vi "Begin.vi"(8 "error in":errorcluster) -> (0 "error out":errorcluster)   [LabVIEW 2014]
doc: "Called before other user functions, this VI is expected to open initial I/O refnums, load in file data, and do all program initialization. Notice that the <B>error out</B> terminal is simply used for data flow. Wiring it to other structures or subVIs ensures that this VI runs first."
uses:
  <vilib>/Rock Robotics/SystemInterfaces/DIO/FPGA_DIOPWMChannel.ctl
  <vilib>/Rock Robotics/WPI/SafetyOutput/WPI_SafetyOutputConfigMenu.ctl
  <vilib>/Rock Robotics/WPI/DriverStation/WPI_DriverStationRobotMode2.ctl
  <vilib>/Rock Robotics/WPI/Joystick/WPI_JoystickDeviceEnum.ctl
  <vilib>/Rock Robotics/WPI/Solenoid/WPI_SolenoidChannel.ctl
  <vilib>/Rock Robotics/SystemInterfaces/DIO/FPGA_DIOChannel.ctl
  <vilib>/Rock Robotics/WPI/Encoder/WPI_EncoderType.ctl
  <vilib>/Rock Robotics/SystemInterfaces/AI/FPGA_AIGyroChannel.ctl
  <vilib>/Rock Robotics/SystemInterfaces/Typedef/FPGA_TypedefAnalogModule.ctl
  <vilib>/Rock Robotics/SystemInterfaces/AI/FPGA_AIChannel.ctl
  <vilib>/Rock Robotics/SystemInterfaces/Typedef/FPGA_TypedefDigitalModule.ctl
  <vilib>/Rock Robotics/SystemInterfaces/Typedef/FPGA_TypedefAnalogModuleForGyro.ctl
  <vilib>/Rock Robotics/WPI/RobotDrive/WPI_RobotDriveOpen2MotorWithTalon.vi
  Robot Global Data.vi
  <vilib>/Rock Robotics/Network Tables/SD Write String Array.vi
  <vilib>/Rock Robotics/WPI/MotorControl/WPI_MotorControlOpen Victor.vi
  <vilib>/Rock Robotics/WPI/Solenoid/WPI_SolenoidOpenDouble.vi
  <vilib>/Rock Robotics/WPI/Counter/WPI_CounterDigitalInputToDigitalSource.vi
  <vilib>/Rock Robotics/WPI/Switch/WPI_SwitchOpenLimit.vi
  <vilib>/Rock Robotics/WPI/Accelerometer/InternalAccelerometer/WPI_AccelerometerInternalOpen.vi
  <vilib>/Rock Robotics/WPI/Camera/WPI_CameraDevRef.ctl
  <vilib>/Rock Robotics/WPI/Ultrasonic/WPI_SonarMB1010AnalogOpen.vi
  <vilib>/Rock Robotics/WPI/Ultrasonic/WPI_SonarMB1010AnalogRefNum Registry Set.vi
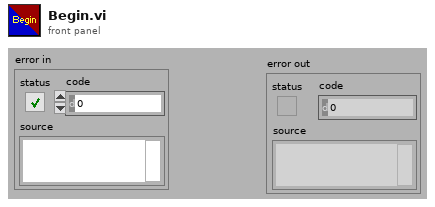
[diagram p1: front panel]
types:
  T1 = typedef "FPGA_TypedefAnalogModuleForGyro.ctl" = enum16{"Controller 1"}
  T2 = typedef "FPGA_AIGyroChannel.ctl" = enum8{"AI 0", "AI 1", "Invalid"}
  T3 = typedef "FPGA_AIChannel.ctl" = enum8{"AI 0", "AI 1", "AI 2", "AI 3", "AI MXP 0", "AI MXP 1", "AI MXP 2", "AI MXP 3", "Invalid"}
  T4 = typedef "FPGA_TypedefAnalogModule.ctl" = enum16{"Controller 1"}
  T5 = typedef "FPGA_TypedefDigitalModule.ctl" = enum16{"Controller 1"}
  T6 = typedef "WPI_EncoderType.ctl" = enum16{"1x", "2x", "4x"}
  T7 = typedef "FPGA_DIOChannel.ctl" = enum8{"DIO 0", "DIO 1", "DIO 2", "DIO 3", "DIO 4", "DIO 5", "DIO 6", "DIO 7", "DIO 8", "DIO 9", "DIO MXP 0", "DIO MXP 1", "DIO MXP 2", "DIO MXP 3", "DIO MXP 4", "DIO MXP 5", "DIO MXP 6", "DIO MXP 7", "DIO MXP 8", "DIO MXP 9", "DIO MXP 10", "DIO MXP 11", "DIO MXP 12", "DIO MXP 13", "DIO MXP 14", "DIO MXP 15", "Invalid"}
  T8 = typedef "WPI_SolenoidChannel.ctl" = enum8{"Solenoid 0", "Solenoid 1", "Solenoid 2", "Solenoid 3", "Solenoid 4", "Solenoid 5", "Solenoid 6", "Solenoid 7", "Invalid"}
  T9 = typedef "FPGA_DIOPWMChannel.ctl" = enum8{"PWM 0", "PWM 1", "PWM 2", "PWM 3", "PWM 4", "PWM 5", "PWM 6", "PWM 7", "PWM 8", "PWM 9", "PWM MXP 0", "PWM MXP 1", "PWM MXP 2", "PWM MXP 3", "PWM MXP 4", "PWM MXP 5", "PWM MXP 6", "PWM MXP 7", "PWM MXP 8", "PWM MXP 9", "Invalid"}
  T10 = typedef "WPI_JoystickDeviceEnum.ctl" = enum16{"USB 0", "USB 1", "USB 2", "USB 3", "USB 4", "USB 5"}
  T11 = typedef "WPI_DriverStationRobotMode2.ctl" = enum16{"Autonomous Disabled", "Autonomous Enabled", "Teleop Disabled", "Teleop Enabled", "Disconnected", "Finish", "Test Disabled", "Test Enabled", "Emergency Stopped"}
  T12 = typedef "WPI_SafetyOutputConfigMenu.ctl" = enum16{"Enable", "Disable"}
  T13 = typedef "WPI_CameraDevRef.ctl" = cluster{"Camera Address":string, "CameraStatus":errorcluster}
  T14 = typedef "WPI_PotentiometerDevRef.ctl" = cluster{"DevStatus":errorcluster, "Controller":T4, "Analog Channel":T3, "Invert Output":bool}
  T15 = typedef "WPI_GyroDevRef.ctl" = cluster{"DevStatus":errorcluster, "Analog Module":T4, "Analog Channel":T3, "Offset":dbl, "Gain (VoltsPerDegree/Second)":dbl}
  T16 = typedef "WPI_JoystickDevRef.ctl" = cluster{"Device":T10}
  T17 = typedef "WPI_RobotDriveDevRef.ctl" = cluster{"DevStatus":errorcluster, "Motors[]":T18[], "Square Inputs":bool, "Max Output":dbl}
  T18 = typedef "WPI_MotorControlDeviceRef.ctl" = cluster{"DeviceStatus":errorcluster, "Type":T19, "PWM":cluster{"Controller":T5, "PWM Channel":T9, "DeadBand":T20}, "CAN":cluster{"Device Number":u8, "Control Mode":T21, "Semaphore":T22, "Max Vout":dbl, "TalonSRX Control Mode":T23}, "Invert":bool, "TransformRef":T24, "InvTransformRef":T24}
  T19 = typedef "WPI_MotorControlType.ctl" = enum16{"PWM", "CAN", "CANTalonSRX"}
  T20 = typedef "WPI_PWMDeadband.ctl" = cluster{"Name":string, "maxPositivePwm":i32, "minPositivePwm":i32, "centerPwm":i32, "maxNegativePwm":i32, "minNegativePwm":i32, "angularRange":u16}
  T21 = typedef "WPI_CANJaguar_ControlMode.ctl" = enum8{"Percent VBus", "Current", "Speed", "Position", "Voltage"}
  T22 = typedef "Semaphore RefNum" = refnum<k1>
  T23 = typedef "WPI_CANTalonSRX_APIControlMode.ctl" = enum8{"Percent VBus", "Speed", "Position", "Slave", "Unchanged / Invalid"}
  T24 = typedef "WPI_PWMTransform_ConPane.ctl" = refnum<vi>
  T25 = typedef "WPI_DigitalInputDevRef.ctl" = cluster{"DevStatus":errorcluster, "DIO Channel":T7, "Controller":T5}
  T26 = typedef "FPGA_CounterEncoderSourceConvertionLVSourceType.ctl" = cluster{"DevStatus":errorcluster, "AnalogTriggerMode?":bool, "DigitalMode":cluster{"Controller":T5, "DIO Channel":T27}, "AnalogTriggerMode":cluster{"AnalogTriggerIndex":T28, "OutputType":T29}}
  T27 = typedef "FPGA_DIODigitalSourceChannel.ctl" = enum8{"DIO 0", "DIO 1", "DIO 2", "DIO 3", "DIO 4", "DIO 5", "DIO 6", "DIO 7", "DIO 8", "DIO 9", "DIO MXP 0", "DIO MXP 1", "DIO MXP 2", "DIO MXP 3", "DIO MXP 4", "DIO MXP 5", "DIO MXP 6", "DIO MXP 7", "DIO MXP 8", "DIO MXP 9", "DIO MXP 10", "DIO MXP 11", "DIO MXP 12", "DIO MXP 13", "DIO MXP 14", "DIO MXP 15", "Disabled"}
  T28 = typedef "FPGA_AnalogTriggerIndex.ctl" = enum8{"Trig 0", "Trig 1", "Trig 2", "Trig 3", "Trig 4", "Trig 5", "Trig 6", "Trig 7", "Invalid"}
  T29 = typedef "FPGA_AnalogTriggerOutType.ctl" = enum16{"InWindow", "TriggerState", "Rising", "Falling"}
  T30 = typedef "WPI_EncoderDevRef.ctl" = cluster{"DevStatus":errorcluster, "EncoderIndex":T31, "CounterIndex":T32, "DistancePerCount":dbl, "Decoding Type":T6}
  T31 = typedef "FPGA_EncoderIdx.ctl" = enum8{"Enc 0", "Enc 1", "Enc 2", "Enc 3", "Enc 4", "Enc 5", "Enc 6", "Enc 7", "Invalid"}
  T32 = typedef "FPGA_CounterCtrSystemIndex.ctl" = enum8{"Ctr 0", "Ctr 1", "Ctr 2", "Ctr 3", "Ctr 4", "Ctr 5", "Ctr 6", "Ctr 7", "Invalid"}
  T33 = typedef "WPI_AccelerometerDevRef.ctl" = cluster{"DevStatus":errorcluster, "Controller":T4, "Scaling":T34, "Analog Channels":T35, "I2C Bus":T36, "SPI Bus":T37, "Accel Range":T38, "ADXL345 Axes":T39, "Handle":i32, "Device Address":u8, "Accel Type":enum16{"Analog", "ADXL345 I2C", "ADXL345 SPI", "Internal"}}
  T34 = typedef "WPI_AccelerometerScaling.ctl" = cluster{"Gain (VoltsPerG)":dbl, "Center Voltage":dbl}
  T35 = typedef "WPI_AccelerometerAnalogChannels.ctl" = cluster{"X-Axis":T3, "Y-Axis":T3, "Z-Axis":T3}
  T36 = typedef "i2c_bus.ctl" = enum16{"I2C On-Board", "I2C MXP", "Invalid"}
  T37 = typedef "spi_bus.ctl" = enum16{"SPI On-Board, CS0", "SPI On-Board, CS1", "SPI On-Board, CS2", "SPI On-Board, CS3", "SPI MXP", "Invalid"}
  T38 = typedef "ADXL345 Range.ctl" = u8
  T39 = typedef "WPI_AccelerometerADXL345 Axes.ctl" = cluster{"X-Axis":bool, "Y-Axis":bool, "Z-Axis":bool}
  T40 = typedef "WPI_SwitchDevRef.ctl" = cluster{"DevStatus":errorcluster, "DIO Channel":T7, "Controller":T5, "CntIndex":T32, "Normally Closed":bool}
  T41 = typedef "WPI_SonarMB1010AnalogDeviceRef.ctl" = cluster{"AIDeviceRef":T42, "Scaling factor (V/in)":dbl, "Average Bits":u8}
  T42 = typedef "WPI_AnalogChannelDevRef.ctl" = cluster{"DevStatus":errorcluster, "Controller":T4, "Analog Channel":T3}
  T43 = typedef "WPI_SolenoidDevRef.ctl" = cluster{"DevStatus":errorcluster, "Pneumatics Control Module":u8, "Forward Solenoid Channel":T8, "Reverse Solenoid Channel":T8}
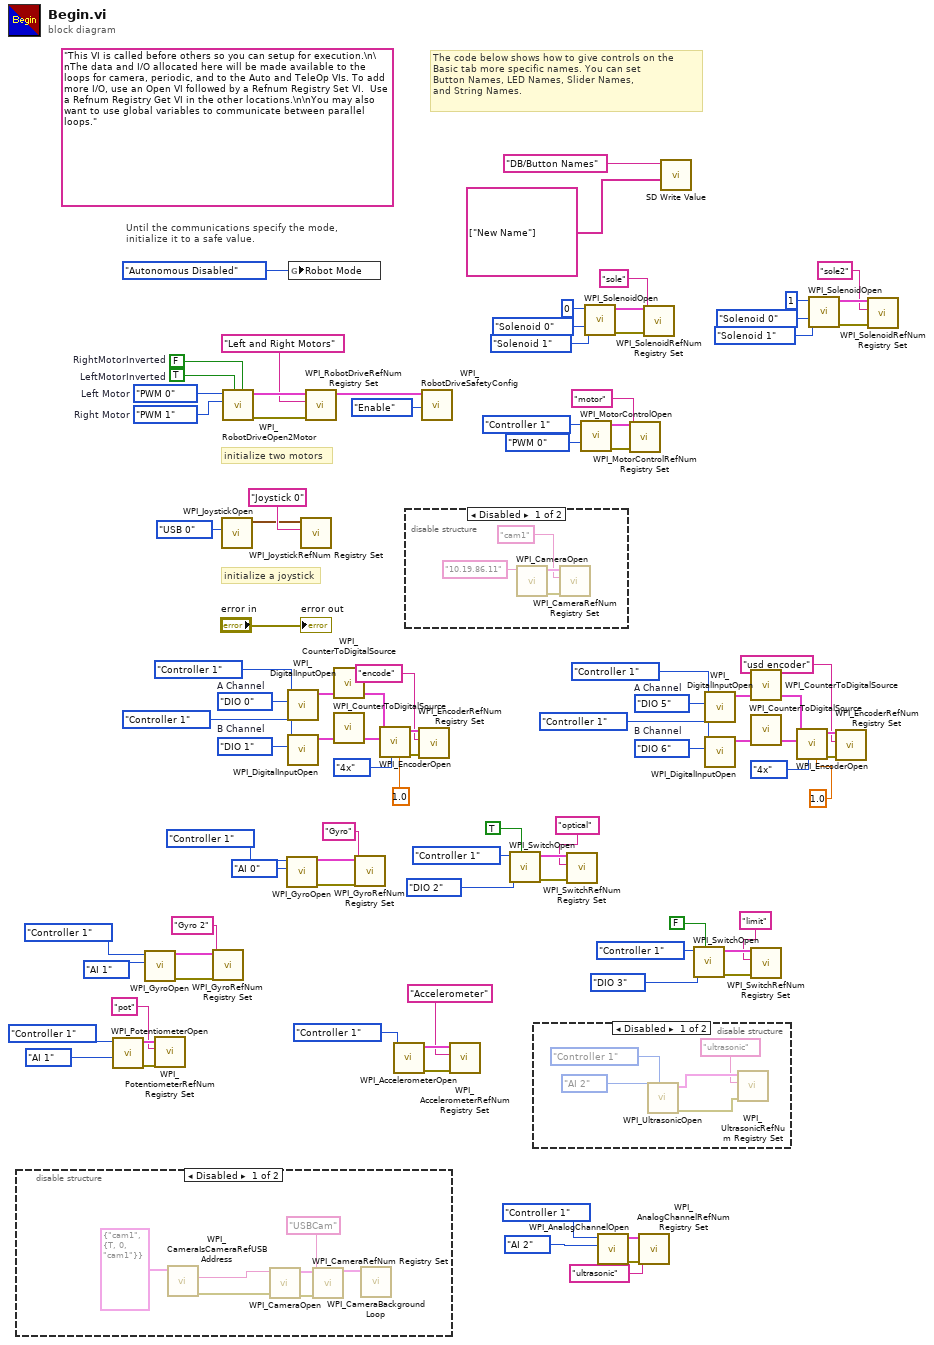
[diagram p0: block diagram]
diagram:
  w23 = FPGA_DIOChannel."DIO 6"  # B Channel
  w22 = FPGA_DIOChannel."DIO 5"  # A Channel
  w62 = FPGA_DIOChannel."DIO 1"  # B Channel
  w61 = FPGA_DIOChannel."DIO 0"  # A Channel
  (unwired) "This VI is called before others so you can setup for execution.\n\nThe data and I/O allocated here will be made available to the loops for camera, periodic, and to the Auto and TeleOp VIs. To add more I/O, use an Open VI followed by a Refnum Registry Set VI.  Use a Refnum Registry Get VI in the other locations.\n\nYou may also want to use global variables to communicate between parallel loops."
  w89 = FPGA_DIOPWMChannel."PWM 1"  # Right Motor
  w90 = FPGA_DIOPWMChannel."PWM 0"  # Left Motor
  w94 = TRUE  # LeftMotorInverted
  w95 = FALSE  # RightMotorInverted
  # "The code below shows how to give controls on the\nBasic tab more specific names. You can set\nButton Names, LED Names, Slider Names,\nand String Names."
  # "initialize a joystick"
  # "Until the communications specify the mode,\ninitialize it to a safe value."
  # "initialize two motors"
  n1 = disable-structure shown="Disabled" {
    frame Disabled {
      n2 = call <vilib>:"WPI_CameraIsCameraRefUSBAddress.vi"("CameraDevRef"=T13 {"Camera Address"="cam1", "CameraStatus"={"status"=TRUE, "code"=0, "source"="cam1"}}) -> ("error out"=w98:errorcluster, "Camera Address Out"=w99:string)  [unwired: 7 in, 2 out]
      n3 = call <vilib>:"WPI_CameraOpen.vi"("error in (no error)"=w98, "Camera Address"=w99) -> ("error out"=w100:errorcluster, "CameraDevRef"=w101:T13)  [unwired: 8 in]
      n4 = call <vilib>:"WPI_CameraRefNum Registry Set.vi"("error in (no error)"=w100, "refnum name"="USBCam", "CameraDevRef"=w101) -> ("CameraDevRef"=w97:T13)  [unwired: 7 in, 1 out]
      n5 = call <vilib>:"WPI_CameraBackground Loop.vi"("CameraDevRef"=w97) -> ()  [unwired: 11 in]
    }
    frame Enabled {
    }
  }
  n6 = call <vilib>:"WPI_PotentiometerOpen.vi"("Analog Channel"=FPGA_AIChannel."AI 1", "Controller"=FPGA_TypedefAnalogModule."Controller 1") -> ("error out"=w42:errorcluster, "PotDevRef"=w41:T14)  [unwired: 8 in]
  n7 = call <vilib>:"WPI_GyroOpen.vi"("Analog Channel"=FPGA_AIGyroChannel."AI 1", "Controller"=FPGA_TypedefAnalogModuleForGyro."Controller 1") -> ("error out"=w5:errorcluster, "GyroDevRef"=w3:T15)  [unwired: 7 in, 1 out]
  n8 = call <vilib>:"WPI_PotentiometerRefNum Registry Set.vi"("error in (no error)"=w42, "refnum name"="pot", "PotDevRef"=w41) -> ()  [unwired: 7 in, 2 out]
  n9 = call <vilib>:"WPI_GyroRefNum Registry Set.vi"("error in (no error)"=w5, "refnum name"="Gyro 2", "GyroDevRef"=w3) -> ()  [unwired: 7 in, 2 out]
  n10 = call <vilib>:"WPI_JoystickOpen.vi"("JoystickDevice"=WPI_JoystickDeviceEnum."USB 0") -> ("JoystickDevRef"=w84:T16)  [unwired: 10 in]
  n11 = call-poly <vilib>:"WPI_RobotDriveOpen2Motor.vi"("Right Motor Inverted"=w95, "Left Motor Inverted"=w94, "Right Motor"=w89, "Left Motor"=w90) -> ("error out"=w91:errorcluster, "RobotDriveDevRef"=w93:T17)  [unwired: 1 in, 5 out]
  n12 = call <vilib>:"WPI_GyroOpen.vi"("Analog Channel"=FPGA_AIGyroChannel."AI 0", "Controller"=FPGA_TypedefAnalogModuleForGyro."Controller 1") -> ("error out"=w49:errorcluster, "GyroDevRef"=w47:T15)  [unwired: 7 in, 1 out]
  n13 = call <vilib>:"WPI_DigitalInputOpen.vi"("DIO Channel"=w61, "Controller"=FPGA_TypedefDigitalModule."Controller 1") -> ("DigitalInputDevRef"=w58:T25)  [unwired: 1 in, 8 out]
  n14 = call <vilib>:"WPI_DigitalInputOpen.vi"("DIO Channel"=w62, "Controller"=FPGA_TypedefDigitalModule."Controller 1") -> ("DigitalInputDevRef"=w59:T25)  [unwired: 1 in, 8 out]
  n15 = global write "Robot Global Data.vi" "Robot Mode"(WPI_DriverStationRobotMode2."Autonomous Disabled" ("Robot Mode")) -> ()
  n16 = call <vilib>:"WPI_JoystickRefNum Registry Set.vi"("refnum name"="Joystick 0", "JoystickDevRef"=w84) -> ()  [unwired: 8 in, 2 out]
  n17 = call <vilib>:"WPI_RobotDriveRefNum Registry Set.vi"("error in (no error)"=w91, "refnum name"="Left and Right Motors", "RobotDriveDevRef"=w93) -> ("RobotDriveDevRef"=w88:T17)  [unwired: 8 out]
  n18 = call-poly <vilib>:"WPI_CounterToDigitalSource.vi"("DigitalInputDevRef"=w58) -> ("Digital Source"=w57:T26)  [unwired: 6 out]
  n19 = call-poly <vilib>:"WPI_CounterToDigitalSource.vi"("DigitalInputDevRef"=w59) -> ("Digital Source"=w60:T26)  [unwired: 6 out]
  n20 = call <vilib>:"WPI_GyroRefNum Registry Set.vi"("error in (no error)"=w49, "refnum name"="Gyro", "GyroDevRef"=w47) -> ()  [unwired: 7 in, 2 out]
  n21 = call <vilib>:"WPI_EncoderOpen.vi"("DistancePerCount"=1.0, "Decoding Type"=WPI_EncoderType."4x", "BSource"=w60, "ASource"=w57) -> ("error out"=w56:errorcluster, "EncoderDevRef"=w55:T30)  [unwired: 4 in, 2 out]
  n22 = call-poly <vilib>:"WPI_AccelerometerOpen.vi"("Controller"=FPGA_TypedefAnalogModule."Controller 1") -> ("error out"=w27:errorcluster, "AccelerometerDevRef"=w26:T33)  [unwired: 9 in]
  n23 = disable-structure shown="Disabled" {
    frame Disabled {
      n24 = call <vilib>:"WPI_CameraOpen.vi"("Camera Address"="10.19.86.11") -> ("error out"=w106:errorcluster, "CameraDevRef"=w105:T13)  [unwired: 9 in]
      n25 = call <vilib>:"WPI_CameraRefNum Registry Set.vi"("error in (no error)"=w106, "refnum name"="cam1", "CameraDevRef"=w105) -> ()  [unwired: 7 in, 2 out]
    }
    frame Enabled {
    }
  }
  n26 = call <vilib>:"WPI_EncoderRefNum Registry Set.vi"("error in (no error)"=w56, "refnum name"="encode", "EncoderDevRef"=w55) -> ()  [unwired: 7 in, 2 out]
  n27 = call <vilib>:"WPI_RobotDriveSafetyConfig.vi"("mode"=WPI_SafetyOutputConfigMenu."Enable", "RobotDriveDevRef"=w88) -> ()  [unwired: 8 in, 2 out]
  n28 = call <vilib>:"WPI_AccelerometerRefNum Registry Set.vi"("error in (no error)"=w27, "refnum name"="Accelerometer", "AccelerometerDevRef"=w26) -> ()  [unwired: 7 in, 2 out]
  n29 = call-poly <vilib>:"WPI_SwitchOpen.vi"("Normally Closed"=TRUE, "DIO Channel"=FPGA_DIOChannel."DIO 2", "Controller"=FPGA_TypedefDigitalModule."Controller 1") -> ("error out"=w38:errorcluster, "SwitchDevRef"=w39:T40)  [unwired: 7 in]
  n30 = disable-structure shown="Disabled" {
    frame Disabled {
      n31 = call-poly <vilib>:"WPI_UltrasonicOpen.vi"("Controller"=FPGA_TypedefAnalogModule."Controller 1", "Analog Channel"=FPGA_AIChannel."AI 2") -> ("error out"=w110:errorcluster, "SonarMB1010AnalogDevRef"=w111:T41)  [unwired: 8 in]
      n32 = call-poly <vilib>:"WPI_UltrasonicRefNum Registry Set.vi"("error in (no error)"=w110, "refnum name"="ultrasonic", "SonarMB1010AnalogDevRef"=w111) -> ()  [unwired: 7 in, 2 out]
    }
    frame Enabled {
    }
  }
  n33 = call <vilib>:"WPI_SwitchRefNum Registry Set.vi"("error in (no error)"=w38, "refnum name"="optical", "SwitchDevRef"=w39) -> ()  [unwired: 7 in, 2 out]
  n34 = call-poly <vilib>:"WPI_MotorControlOpen.vi"("PWM Channel"=FPGA_DIOPWMChannel."PWM 0", "Controller"=FPGA_TypedefDigitalModule."Controller 1") -> ("error out"=w74:errorcluster, "MotorControlDeviceRef"=w73:T18)  [unwired: 8 in]
  n35 = call-poly <vilib>:"WPI_SolenoidOpen.vi"("Reverse Solenoid Channel"=WPI_SolenoidChannel."Solenoid 1", "Forward Solenoid Channel"=WPI_SolenoidChannel."Solenoid 0" ("Solenoid Channel"), "Pneumatics Control Module (0)"=u8 0) -> ("error out"=w79:errorcluster, "SolenoidDevRef"=w78:T43)  [unwired: 7 in]
  n36 = call <vilib>:"WPI_AnalogChannelOpen.vi"("Analog Channel"=FPGA_AIChannel."AI 2", "Controller"=FPGA_TypedefAnalogModule."Controller 1") -> ("error out"=w8:errorcluster, "AIDeviceRef"=w7:T42)  [unwired: 8 in]
  n37 = call <vilib>:"WPI_MotorControlRefNum Registry Set.vi"("error in (no error)"=w74, "refnum name"="motor", "MotorControlDevRef"=w73) -> ()  [unwired: 7 in, 2 out]
  n38 = call <vilib>:"WPI_AnalogChannelRefNum Registry Set.vi"("error in (no error)"=w8, "refnum name"="ultrasonic", "AIDeviceRef"=w7) -> ()  [unwired: 7 in, 2 out]
  n39 = call <vilib>:"WPI_SolenoidRefNum Registry Set.vi"("error in (no error)"=w79, "refnum name"="sole", "SolenoidDevRef"=w78) -> ()  [unwired: 7 in, 2 out]
  n40 = call-poly <vilib>:"SD Write Value.vi"("String Array"=string[] ["New Name"], "Name"="DB/Button Names") -> ()  [unwired: 8 in, 2 out]
  n41 = call-poly <vilib>:"WPI_SwitchOpen.vi"("Normally Closed"=FALSE, "DIO Channel"=FPGA_DIOChannel."DIO 3", "Controller"=FPGA_TypedefDigitalModule."Controller 1") -> ("error out"=w32:errorcluster, "SwitchDevRef"=w33:T40)  [unwired: 7 in]
  n42 = call <vilib>:"WPI_DigitalInputOpen.vi"("DIO Channel"=w22, "Controller"=FPGA_TypedefDigitalModule."Controller 1") -> ("DigitalInputDevRef"=w19:T25)  [unwired: 1 in, 8 out]
  n43 = call <vilib>:"WPI_DigitalInputOpen.vi"("DIO Channel"=w23, "Controller"=FPGA_TypedefDigitalModule."Controller 1") -> ("DigitalInputDevRef"=w20:T25)  [unwired: 1 in, 8 out]
  n44 = call-poly <vilib>:"WPI_CounterToDigitalSource.vi"("DigitalInputDevRef"=w19) -> ("Digital Source"=w18:T26)  [unwired: 6 out]
  n45 = call-poly <vilib>:"WPI_CounterToDigitalSource.vi"("DigitalInputDevRef"=w20) -> ("Digital Source"=w21:T26)  [unwired: 6 out]
  n46 = call <vilib>:"WPI_SwitchRefNum Registry Set.vi"("error in (no error)"=w32, "refnum name"="limit", "SwitchDevRef"=w33) -> ()  [unwired: 7 in, 2 out]
  n47 = call <vilib>:"WPI_EncoderOpen.vi"("DistancePerCount"=1.0, "Decoding Type"=WPI_EncoderType."4x", "BSource"=w21, "ASource"=w18) -> ("error out"=w17:errorcluster, "EncoderDevRef"=w16:T30)  [unwired: 4 in, 2 out]
  n48 = call-poly <vilib>:"WPI_SolenoidOpen.vi"("Reverse Solenoid Channel"=WPI_SolenoidChannel."Solenoid 1", "Forward Solenoid Channel"=WPI_SolenoidChannel."Solenoid 0" ("Solenoid Channel"), "Pneumatics Control Module (0)"=u8 1) -> ("error out"=w68:errorcluster, "SolenoidDevRef"=w67:T43)  [unwired: 7 in]
  n49 = call <vilib>:"WPI_EncoderRefNum Registry Set.vi"("error in (no error)"=w17, "refnum name"="usd encoder", "EncoderDevRef"=w16) -> ()  [unwired: 7 in, 2 out]
  n50 = call <vilib>:"WPI_SolenoidRefNum Registry Set.vi"("error in (no error)"=w68, "refnum name"="sole2", "SolenoidDevRef"=w67) -> ()  [unwired: 7 in, 2 out]
  "error out" <- "error in"
